vi "Operate.vi"(0 "Subtract in":refnum<class "Subtract.lvclass">, 11 "error in (no error)":errorcluster) -> (4 "Subtract out":refnum<class "Subtract.lvclass">, 15 "error out":errorcluster)   [LabVIEW 2020, in "Subtract.lvclass"]
uses:
  Subtract.lvclass
  C:/Users/khishore.kumar/Khishore/labview_tips_2024/src/Assignment 25/Arithmetic Operations/Arithmetic Operations.lvclass
  Arithmetic Operations.lvclass/Arithmetic Operations.ctl
  Accessors/Read/Read A.vi
  Accessors/Read/Read B.vi
  Accessors/Write/Write C.vi
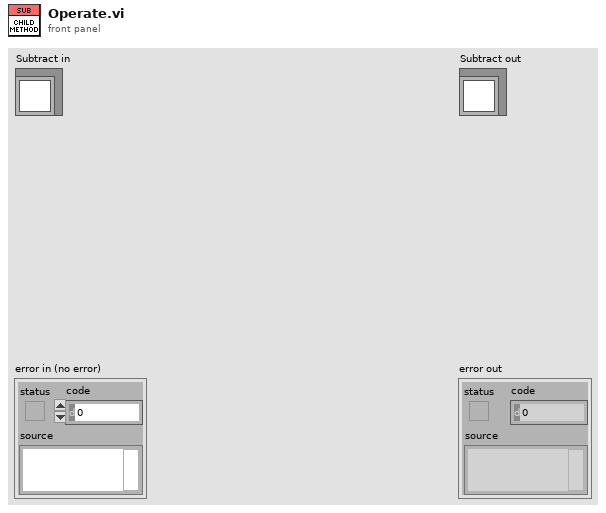
[diagram p1: front panel]
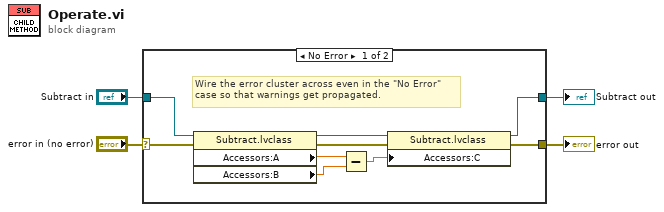
[diagram p0: block diagram]
diagram:
  n1 = case shown="No Error" "error in (no error)" {
    selector: "error in (no error)" -> [w13 w15]
    tunnel: [w11 w15] -> w3
    tunnel: "Subtract in" -> [w10 w14]
    tunnel: [w5 w14] -> w1
    frame No Error {
      # "Wire the error cluster across even in the \"No Error\"\ncase so that warnings get propagated."
      n2 = property class="Subtract.lvclass"(reference=w10, error in=w13) -> (reference out=w9:refnum<class "Subtract.lvclass">, error out=w12:errorcluster, "Accessors:A"=w6:dbl, "Accessors:B"=w7:dbl)
      n3 = Subtract(x=w6, y=w7) -> (x-y=w8:dbl)
      n4 = property class="Subtract.lvclass"(reference=w9, error in=w12, "Accessors:C"=w8) -> (reference out=w5:refnum<class "Subtract.lvclass">, error out=w11:errorcluster)
    }
    frame Error {
    }
  }
  "error out" <- w3
  "Subtract out" <- w1
